vi "报表标题输入.vi"(8 "错误输入（无错误）":errorcluster caption="error out", 9 "油动机名称":string, 10 "_sheet_name":string, 11 "NI_report输入":refnum<class "NI_report.lvclass">) -> (0 "错误输出":errorcluster caption="error out", 3 "NI_report输出":refnum<class "NI_report.lvclass">)   [LabVIEW 2013]
doc: "报表标题"
uses:
  <vilib>/Utility/NIReport.llb/NI_report.lvclass
  <vilib>/Utility/NIReport.llb/Append Report Text (str wrap).vi
panel:
  out "输出簇":T1
  # "快关L2_油动机试验报告"
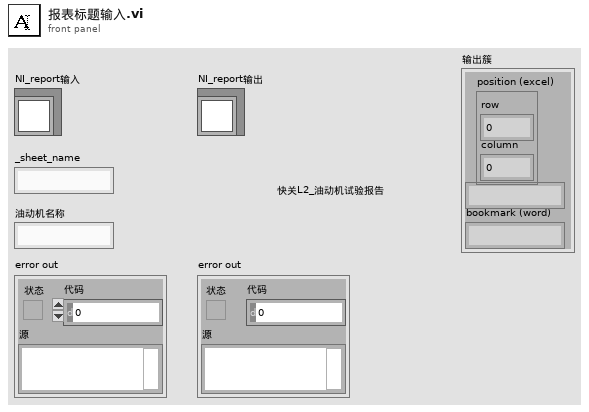
[diagram p1: front panel]
types:
  T1 = cluster{"position (excel)":cluster{"row":i32, "column":i32}, string, "bookmark (word)":string}
  T2 = cluster{"Italic":enum16{"Italic Unchanged", "Italic On", "Italic Off"}, "Strike Through":enum16{"Strike Through Unchanged", "Strike Through On", "Strike Through Off"}, "Underline":enum16{"Underline Unchanged", "Underline On", "Underline Off"}, "Bold":enum16{"Bold Unchanged", "Bold On", "Bold Off"}}
  T3 = cluster{"Charset (-1)":i16, "Weight (-1)":i16, "Name":string, "Size":string}
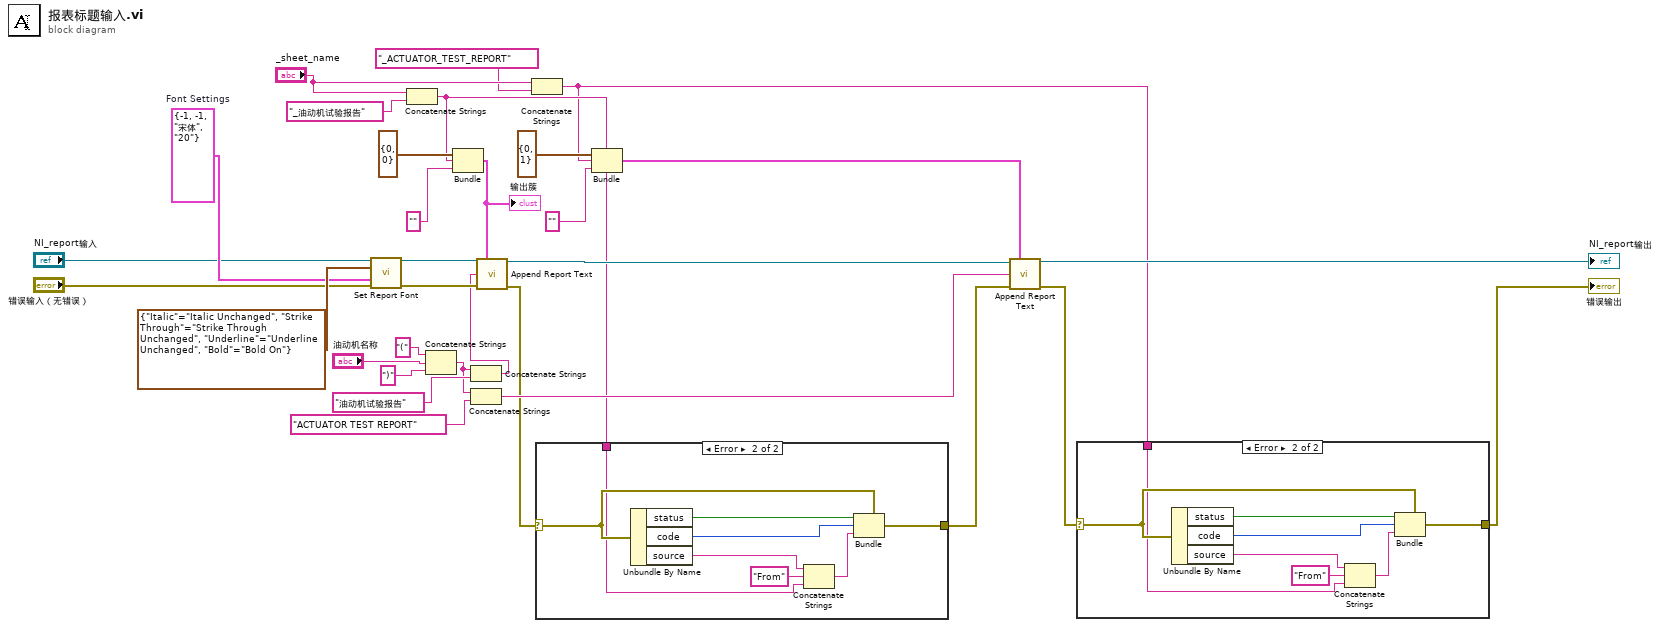
[diagram p0: block diagram]
diagram:
  w15 = T3 {"Charset (-1)"=-1, "Weight (-1)"=-1, "Name"="宋体", "Size"="20"}  # Font Settings
  n1 = call-dynamic "Set Report Font.vi"("report in"="NI_report输入", "text options"=T2 {"Italic"=enum."Italic Unchanged", "Strike Through"=enum."Strike Through Unchanged", "Underline"=enum."Underline Unchanged", "Bold"=enum."Bold On"}, "font settings"=w15, "error in (no error)"="错误输入（无错误）") -> ("report out"=w9:refnum<class "NI_report.lvclass">, "error out"=w10:errorcluster)  [unwired: 9 in, 1 out]
  n2 = Concatenate Strings("_sheet_name", "_油动机试验报告" ("name (excel)")) -> (w5:string)
  n3 = Concatenate Strings("(" ("字符串"), "油动机名称", ")" ("字符串")) -> (w25:string)
  n4 = Bundle("position (excel)"=cluster{"row":i32, "column":i32} {"row"=0, "column"=0}, w5, "bookmark (word)"="") -> (w1:T1)  [unwired: 1 in]
  "输出簇" <- w1
  n5 = Concatenate Strings(w25, "油动机试验报告" ("字符串")) -> (w8:string)
  n6 = Concatenate Strings(w25, "ACTUATOR TEST REPORT" ("字符串")) -> (w30:string)
  n7 = call-poly <vilib>:"Append Report Text.vi"("report in"=w9, "MS Office parameters"=w1, "text"=w8, "error in (no error)"=w10) -> ("report out"=w20:refnum<class "NI_report.lvclass">, "error out"=w7:errorcluster)  [unwired: 8 in, 2 out]
  n8 = Concatenate Strings("_sheet_name", "_ACTUATOR_TEST_REPORT" ("name (excel)")) -> (w2:string)
  n9 = case shown="Error" w7 {
    selector: w7 -> [w32 w39]
    tunnel: [w32 w40] -> w6
    tunnel: w5 -> [_ w34]
    frame No Error {
    }
    frame Error {
      n10 = Unbundle By Name(w39) -> ("status"=w38:bool, "code"=w37:i32, "source"=w35:string)
      n11 = Concatenate Strings(w35, "From", w34) -> (w33:string)
      n12 = Bundle(cluster=w39, "status"=w38, "code"=w37, "source"=w33) -> (w40:errorcluster)
    }
  }
  n13 = Bundle("position (excel)"=cluster{"row":i32, "column":i32} {"row"=0, "column"=1}, w2, "bookmark (word)"="") -> (w19:T1)  [unwired: 1 in]
  n14 = call-poly <vilib>:"Append Report Text.vi"("report in"=w20, "MS Office parameters"=w19, "text"=w30, "error in (no error)"=w6) -> ("report out"=→"NI_report输出":refnum<class "NI_report.lvclass">, "error out"=w3:errorcluster)  [unwired: 8 in, 2 out]
  n15 = case shown="Error" w3 {
    selector: w3 -> [w41 w48]
    tunnel: [w41 w49] -> w4
    tunnel: w2 -> [_ w43]
    frame No Error {
    }
    frame Error {
      n16 = Unbundle By Name(w48) -> ("status"=w47:bool, "code"=w46:i32, "source"=w44:string)
      n17 = Concatenate Strings(w44, "From", w43) -> (w42:string)
      n18 = Bundle(cluster=w48, "status"=w47, "code"=w46, "source"=w42) -> (w49:errorcluster)
    }
  }
  "错误输出" <- w4
